vi "Human Readable Error Message.vi"(3 "error in (no error)":errorcluster) -> (5 "Human readable error message":string)   [LabVIEW 2021, in "CIFCoreCommon.lvlib"]
uses:
  CIFCoreCommon.lvlib
  <vilib>/Utility/error.llb/whitespace.ctl
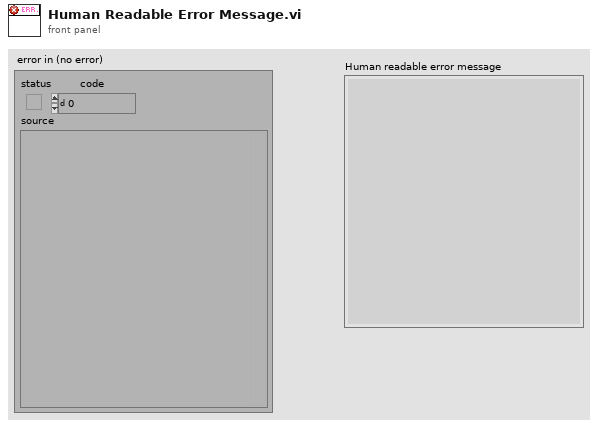
[diagram p1: front panel]
types:
  T1 = typedef "TagReturnType.ctl" = enum16{"No Tag", "<err>", "<append>"}
  T2 = typedef "whitespace.ctl" = u16
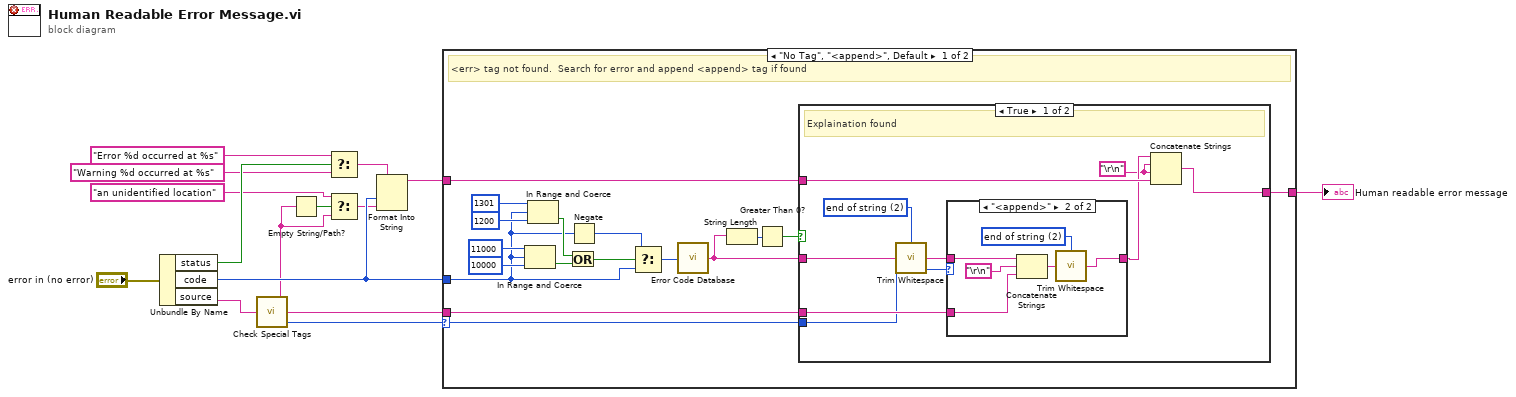
[diagram p0: block diagram]
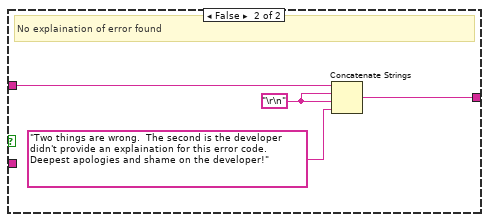
[diagram p3: hidden frame]
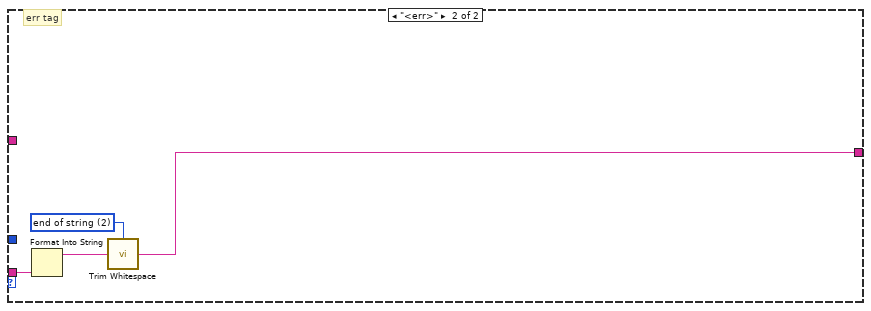
[diagram p4: hidden frame]
diagram:
  n1 = Unbundle By Name("error in (no error)") -> ("status"=w6:bool, "code"=w14:i32, "source"=w15:string)
  n2 = call <vilib>:"Check Special Tags.vi"("source"=w15) -> ("Before Tag (source)"=w8:string, "After Tag (special data)"=w11:string, "Tag Found?"=w7:T1)
  n3 = Empty String/Path?(string/path=w8) -> (empty?=w12:bool)
  n4 = Select(t="Error %d occurred at %s" ("Error %d occurred at %s"), s=w6, f="Warning %d occurred at %s" ("Warning %d occurred at %s")) -> (s? t:f=w10:string)
  n5 = Select(t="an unidentified location" ("an unidentified location"), s=w12, f=w8) -> (s? t:f=w9:string)
  n6 = Format Into String(format string=w10, w14, w9) -> (resulting string=w2:string)  [unwired: 2 in, 1 out]
  n7 = case shown="\"No Tag\", \"<append>\", Default" w7 {
    selector: w7 -> [w20 _]
    tunnel: w14 -> [w21 _]
    tunnel: w11 -> [w23 w55]
    tunnel: w2 -> [w17 _]
    tunnel: [w16 w53] -> w1
    frame "No Tag", "<append>", Default {
      # "<err> tag not found.  Search for error and append <append> tag if found"
      n8 = In Range and Coerce(upper limit=11000, x=w21, lower limit=10000) -> (In Range?=w27:bool)  [unwired: 1 out]
      n9 = In Range and Coerce(upper limit=1301, x=w21, lower limit=1200) -> (In Range?=w28:bool)  [unwired: 1 out]
      n10 = Or(x=w28, y=w27) -> (x .or. y?=w26:bool)
      n11 = Negate(x=w21) -> (-x=w30:i32)
      n12 = Select(t=w30, s=w26, f=w21) -> (s? t:f=w22:i32)
      n13 = call <vilib>:"Error Code Database.vi"("Error Code"=w22) -> ("Error Text"=w18:string)
      n14 = String Length(string=w18) -> (length=w24:i32)
      n15 = Greater Than 0?(x=w24) -> (x > 0?=w19:bool)
      n16 = case shown="True" w19 {
        tunnel: w18 -> [w35 _]
        tunnel: w20 -> [w38 _]
        tunnel: w23 -> [w40 _]
        tunnel: w17 -> [w37 w52]
        tunnel: [w36 w51] -> w16
        frame True {
          w33 = "\r\n" ("End of Line Constant")
          w39 = T2 2 items=["both", "start of string", "end of string"] ("location (both)")
          # "Explaination found"
          n17 = call <vilib>:"Trim Whitespace.vi"("string"=w35, "location (both)"=w39) -> ("trimmed string"=w41:string)
          n18 = case shown="\"<append>\"" w38 {
            tunnel: w41 -> [w42 w48]
            tunnel: [w42 w46] -> w34
            tunnel: w40 -> [_ w44]
            frame "No Tag", Default {
            }
            frame "<append>" {
              w45 = T2 2 items=["both", "start of string", "end of string"] ("location (both)")
              n19 = Concatenate Strings(w48, "\r\n" ("End of Line Constant"), w44) -> (w47:string)
              n20 = call <vilib>:"Trim Whitespace.vi"("string"=w47, "location (both)"=w45) -> ("trimmed string"=w46:string)
            }
          }
          n21 = Concatenate Strings(w34, w33, w33, w37) -> (w36:string)
        }
        frame False {
          w49 = "\r\n" ("End of Line Constant")
          # "No explaination of error found"
          n22 = Concatenate Strings(w52, w49, w49, "Two things are wrong.  The second is the developer didn't provide an explaination for this error code. Deepest apologies and shame on the developer!" ("Error not listed")) -> (w51:string)
        }
      }
    }
    frame "<err>" {
      w54 = T2 2 items=["both", "start of string", "end of string"] ("location (both)")
      # "err tag"
      n23 = Format Into String(w55) -> (resulting string=w56:string)  [unwired: 3 in, 1 out]
      n24 = call <vilib>:"Trim Whitespace.vi"("string"=w56, "location (both)"=w54) -> ("trimmed string"=w53:string)
    }
  }
  "Human readable error message" <- w1
